vi "GetWeeksInfo2.vi"(8 "error in (no error)":errorcluster, 11 "Report DVR":refnum<data-value>) -> (0 "error out":errorcluster, 1 "Available weeks":string, 2 "List of Weeks":u8[](array[numeric]), 3 "Report DVR Out":refnum<data-value>)   [LabVIEW 2017, in "DS_Lib.lvlib" / "SRReportParser.lvlib"]
uses:
  TypeDefs/WeeklyData.ctl
  Modules/Private Controls/Data Raw.ctl
  SRReportParser.lvlib
  Modules/Data Operations.lvlib
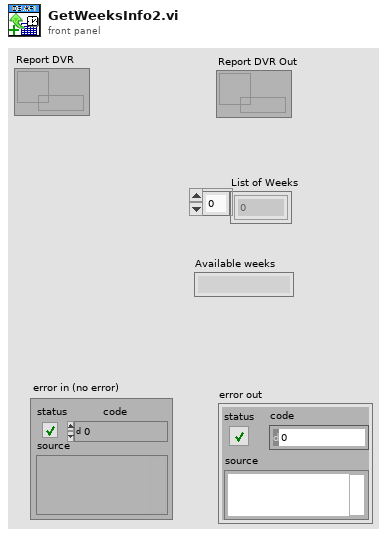
[diagram p1: front panel]
types:
  T1 = typedef "DS_Lib.lvlib/SRReportParser.lvlib/WeeklyData.ctl" = cluster{"Week":u8, "AE-Romania":T2[], "AE-Poland":T2[], "AE-Hungary":T2[], "AE-Czech and Slovakia":T2[]}
  T2 = typedef "Data Operations.lvlib/Data Raw.ctl" = cluster{"SR Number":string, "Status":string, "Summary":string, "AE Owner":string, "AE Group":string, "Contact":string, "SurveyData":cluster{"Resolution Time":dbl, "Total Satisfaction":dbl, "Response Time":dbl, "Courtesy":dbl, "Problem Solved":dbl, "Level of effort":dbl}, "Time Data":cluster{"Last Update Date":timestamp, "Creation Date":timestamp, "Creation week":u8, "Last Update Week":u8}}
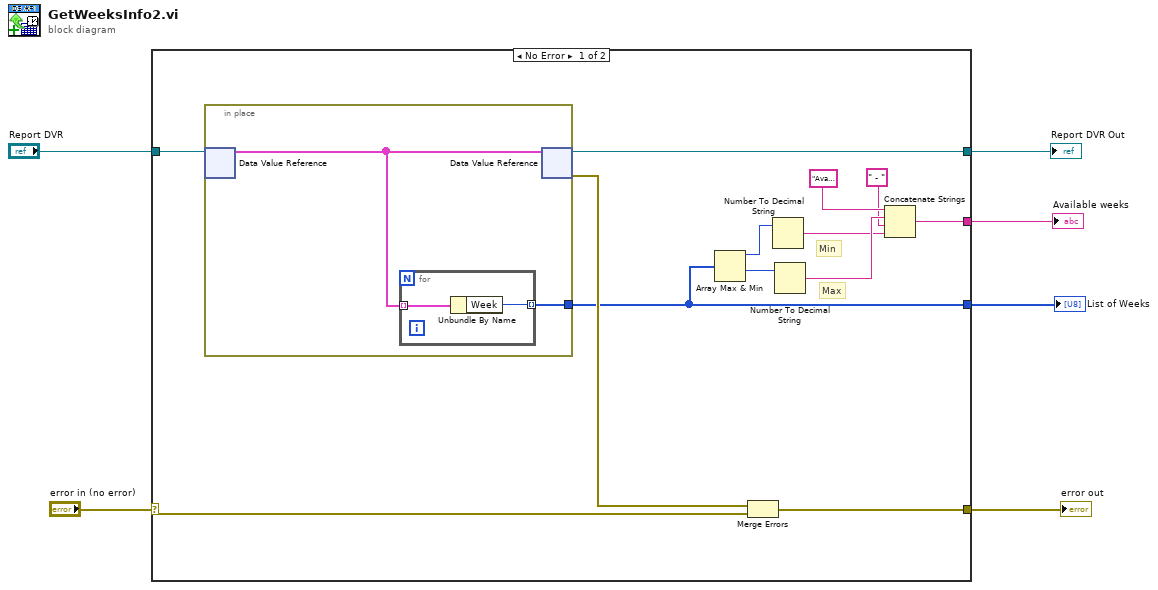
[diagram p0: block diagram]
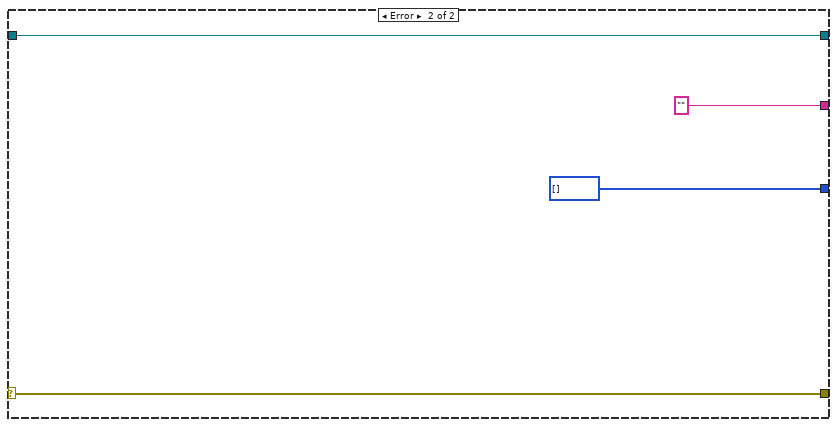
[diagram p2: hidden frame]
diagram:
  n1 = case shown="No Error" "error in (no error)" {
    selector: "error in (no error)" -> [w16 w27]
    tunnel: "Report DVR" -> [w19 w25]
    tunnel: [w17 w27] -> w6
    tunnel: [w11 u8[] []] -> w4
    tunnel: [w15 w25] -> w2
    tunnel: [w7 ""] -> w1
    frame No Error {
      # "Min"
      # "Max"
      n2 = in-place {
        in-place-border: [w21] -> w11
        n3 = in-place-dvr #1(w19) -> (w20:T1[])  [unwired: 1 out]
        n4 = for {
          tunnel: w20 -> [w23] mode=indexing
          tunnel: [w22] -> w21 mode=indexing
          n5 = Unbundle By Name(w23) -> ("Week"=w22:u8)
        }
        n6 = in-place-dvr #1(w20) -> (w15:refnum<data-value>, w18:errorcluster)
      }
      n7 = Array Max & Min(array=w11) -> (max value=w9:u8, min value=w10:u8)  [unwired: 2 out]
      n8 = Merge Errors(w18, w16) -> (w17:errorcluster)
      n9 = Number To Decimal String(number=w9) -> (decimal integer string=w8:string)  [unwired: 1 in]
      n10 = Number To Decimal String(number=w10) -> (decimal integer string=w14:string)  [unwired: 1 in]
      n11 = Concatenate Strings("Available Weeks: ", w14, " - " ("string"), w8) -> (w7:string)
    }
    frame Error {
    }
  }
  "error out" <- w6
  "List of Weeks" <- w4
  "Report DVR Out" <- w2
  "Available weeks" <- w1
